vi "Teleop.vi"(10 "Match Info":T2={"Autonomous Elapsed Seconds"=0.0, "TeleOp Elapsed Seconds"=0.0, "Disabled Elapsed Seconds"=0.0, "Visited Autonomous"=FALSE, "Visited TeleOp"=FALSE, "Visited Disabled"=FALSE, "Autonomous Settings"={"Autonomous Style"=enum."Independent", "VI Refnum"=refnum}}, 11 "Call Context":T3) -> ()   [LabVIEW 2019]
doc: "This VI is called for each TeleOp packet received from the DS where the robot is not disabled. It is often used to read from the joysticks and update I/O or to update setpoints for timed control loops. It should complete and return within 20 milliseconds or it may miss DS packets."
uses:
  <vilib>/Rock Robotics/WPI/DriverStation/WPI_DriverStationDerivedRobotMode.ctl
  <vilib>/Rock Robotics/WPI/DriverStation/WPI_DriverStationMatch Info.ctl
  <vilib>/Rock Robotics/WPI/ThirdParty/Phoenix-LabVIEW/Motor Controller/Controls/CTRE_Phoenix_MotorControl_ControlMode.ctl
  <vilib>/Rock Robotics/WPI/Utilities/WPI_GetSetVariantRefNum.vi
  <vilib>/Rock Robotics/Network Tables/NT Write Boolean Array.vi
  <vilib>/Rock Robotics/Network Tables/NT Write Numeric Array.vi
  <vilib>/Rock Robotics/Network Tables/NT Read Boolean.vi
  <vilib>/Rock Robotics/Network Tables/NT Read Number.vi
  <vilib>/Rock Robotics/WPI/ThirdParty/Phoenix-LabVIEW/Motor Controller/Get/CTRE_Phoenix_MotorController_IntegratedSensorData_TalonFX.vi
  <vilib>/Rock Robotics/WPI/ThirdParty/Phoenix-LabVIEW/Motor Controller/Get/CTRE_Phoenix_MotorController_GetVoltage.vi
  <vilib>/Rock Robotics/WPI/ThirdParty/Phoenix-LabVIEW/Motor Controller/Get/CTRE_Phoenix_MotorController_GetSelectedSensorData.vi
  <vilib>/Rock Robotics/WPI/ThirdParty/Phoenix-LabVIEW/Motor Controller/Get/CTRE_Phoenix_MotorController_GetSupplyAndStatorCurrent_Enhanced.vi
  <vilib>/Rock Robotics/WPI/ThirdParty/Phoenix-LabVIEW/Motor Controller/Get/CTRE_Phoenix_MotorController_GetTemperature.vi
  <vilib>/Rock Robotics/Network Tables/NT Write Number.vi
  <vilib>/Rock Robotics/Network Tables/NT Write Boolean.vi
  Global 2.vi
  <vilib>/addons/control/pid/NI_PID_pid.lvlib
  <vilib>/addons/control/pid/pid.llb/PID (DBL).vi
panel:
  in  "Acc Voltage":dbl=0.5
  in  "DriveScale":dbl(slide)=0.7556179775280899 min=0.25 max=1.0 step=0.1 scale=0.25..1.0
  in  "Steering Scale":dbl(slide)=0.6418539325842696 min=0.25 max=1.0 step=0.1 scale=0.25..1.0
  in  "channel name(s) in (Untitled)":string[](array[string])
  in  "group name in (Untitled)":string="Velocity Data"
  in  "PID gains":T1={"proportional gain (Kc)"=1.0, "integral time (Ti, min)"=0.01, "derivative time (Td, min)"=0.0} {"derivative time (Td, min)" format="%.3f"; "integral time (Ti, min)" format="%.3f"; "proportional gain (Kc)" format="%.3f"}
  out "Horizontal Angle":dbl
  out "Waveform Chart":i32(graph)
  in  "Output":dbl=17250.0
  out "Output Voltage":dbl
  out "Bus Voltage":dbl
  out "Percent Output":dbl
  out "Velocity (Raw Sensor Units per 100 ms)":i32
  out "Position (Raw Sensor Units)":i32
  out "Stator Current":dbl
  out "Supply Current":dbl
  out "Absolute Position":dbl
  out "Velocity":dbl format="%.2f"
  out "Position":dbl format="%.2f"
  out "Sample Slider 0":dbl(slide) scale=0.0..5.0
  out "Sample Boolean 1":bool
  out "Sample Boolean 0":bool
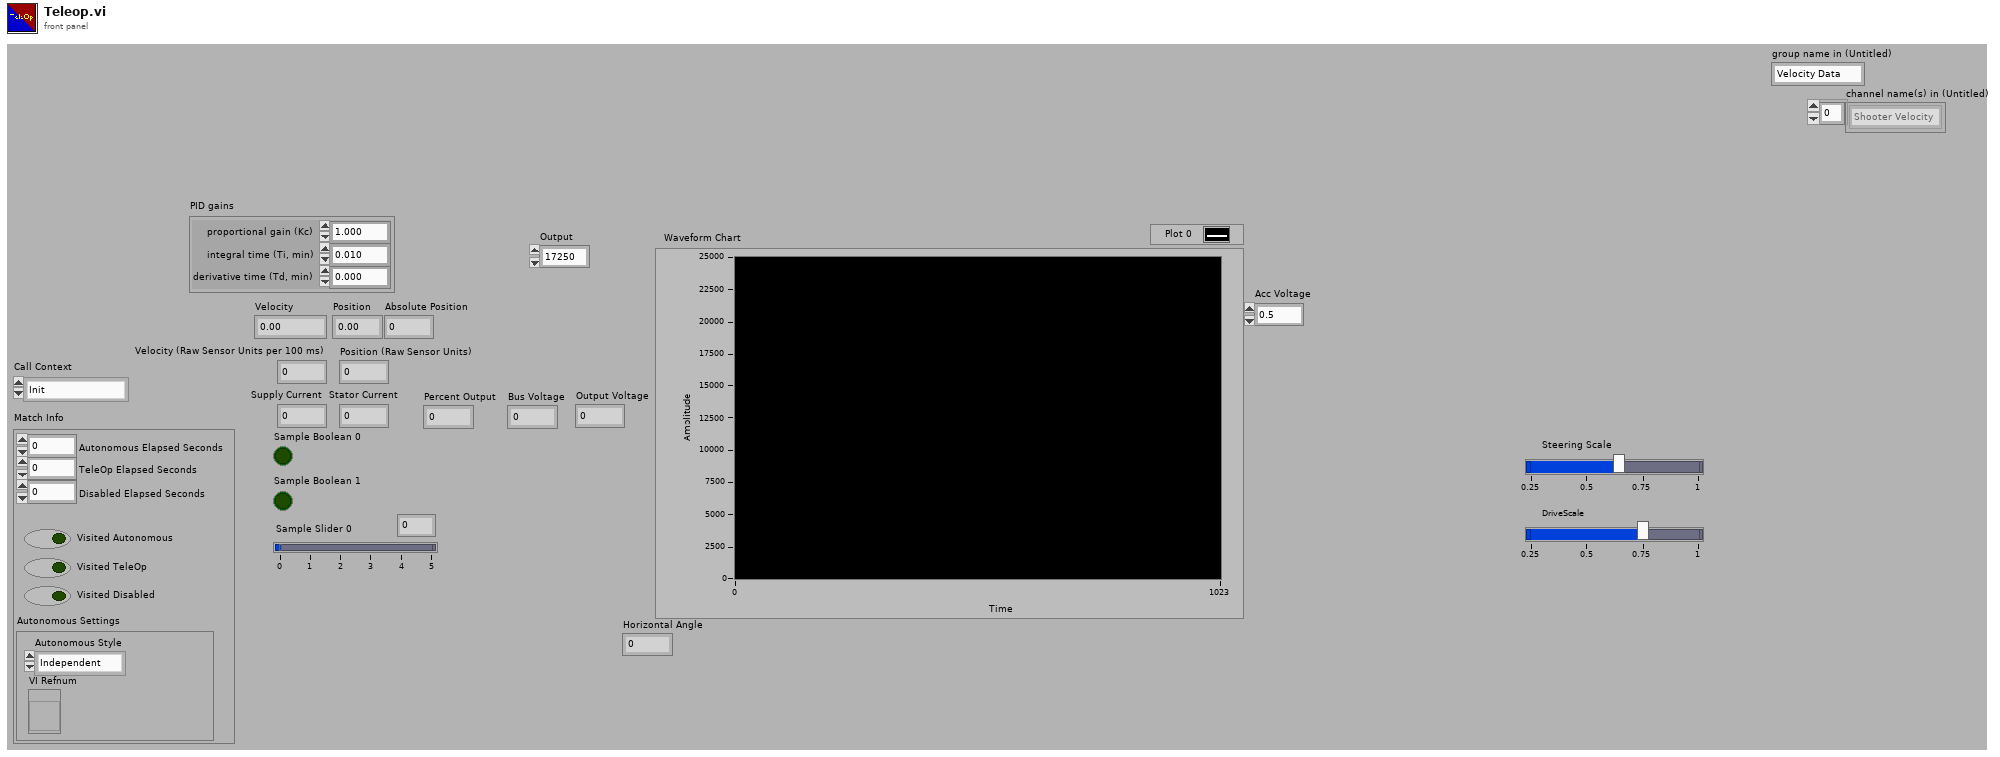
[diagram p1: front panel]
types:
  T1 = cluster{"proportional gain (Kc)":dbl, "integral time (Ti, min)":dbl, "derivative time (Td, min)":dbl}
  T2 = typedef "WPI_DriverStationMatch Info.ctl" = cluster{"Autonomous Elapsed Seconds":dbl, "TeleOp Elapsed Seconds":dbl, "Disabled Elapsed Seconds":dbl, "Visited Autonomous":bool, "Visited TeleOp":bool, "Visited Disabled":bool, "Autonomous Settings":cluster{"Autonomous Style":enum16{"Iterative", "Independent"}, "VI Refnum":refnum<vi>}}
  T3 = typedef "WPI_DriverStationDerivedRobotMode.ctl" = enum16{"Init", "Execute", "Stop"}
  T4 = typedef "CTRE_Phoenix_MotorControl_ControlMode.ctl" = u16
  T5 = typedef "WPI_JoystickDevRef.ctl" = cluster{"Device":T6}
  T6 = typedef "WPI_JoystickDeviceEnum.ctl" = enum16{"USB 0", "USB 1", "USB 2", "USB 3", "USB 4", "USB 5"}
  T7 = cluster{"Axes[0]":dbl, "Axes[1]":dbl, "Axes[2]":dbl, "Axes[3]":dbl, "Axes[4]":dbl, "Axes[5]":dbl, "Axes[6]":dbl, "Axes[7]":dbl, "Axes[8]":dbl}
  T8 = typedef "WPI_MotorControlDeviceRef.ctl" = cluster{"DeviceStatus":errorcluster, "Type":T9, "PWM":cluster{"PWM Channel":T10, "DeadBand":T11}, "CAN":cluster{"Device Number":u8, "SetOutput VI Ref":variant, "GetOutput VI Ref":variant, "Enable VI Ref":variant, "Disable VI Ref":variant, "Data":variant}, "Invert":bool, "DIO PWM":cluster{"PWM \"Enable\" Channel":T10, "DIOChannel":T12, "PWM Rate":dbl}}
  T9 = typedef "WPI_MotorControlType.ctl" = enum16{"PWM", "CAN", "DIO PWM"}
  T10 = typedef "FPGA_DIOPWMChannel.ctl" = enum8{"PWM 0", "PWM 1", "PWM 2", "PWM 3", "PWM 4", "PWM 5", "PWM 6", "PWM 7", "PWM 8", "PWM 9", "PWM MXP 0", "PWM MXP 1", "PWM MXP 2", "PWM MXP 3", "PWM MXP 4", "PWM MXP 5", "PWM MXP 6", "PWM MXP 7", "PWM MXP 8", "PWM MXP 9", "Invalid"}
  T11 = typedef "WPI_PWMDeadband.ctl" = cluster{"Name":string, "maxPositivePwm":i32, "minPositivePwm":i32, "centerPwm":i32, "maxNegativePwm":i32, "minNegativePwm":i32, "angularRange":u16}
  T12 = typedef "FPGA_DIOChannel.ctl" = enum8{"DIO 0", "DIO 1", "DIO 2", "DIO 3", "DIO 4", "DIO 5", "DIO 6", "DIO 7", "DIO 8", "DIO 9", "DIO MXP 0", "DIO MXP 1", "DIO MXP 2", "DIO MXP 3", "DIO MXP 4", "DIO MXP 5", "DIO MXP 6", "DIO MXP 7", "DIO MXP 8", "DIO MXP 9", "DIO MXP 10", "DIO MXP 11", "DIO MXP 12", "DIO MXP 13", "DIO MXP 14", "DIO MXP 15", "SPI Port CS1", "SPI Port CS2", "SPI Port CS3", "SPI Port MISO", "SPI Port MOSI", "Invalid"}
  T13 = cluster{"Buttons[0]":bool, "Buttons[1]":bool, "Buttons[2]":bool, "Buttons[3]":bool, "Buttons[4]":bool, "Buttons[5]":bool, "Buttons[6]":bool, "Buttons[7]":bool, "Buttons[8]":bool}
  T14 = typedef "WPI_RobotDriveDevRef.ctl" = cluster{"DevStatus":errorcluster, "Motors[]":T8[], "Square Inputs":bool, "Max Output":dbl}
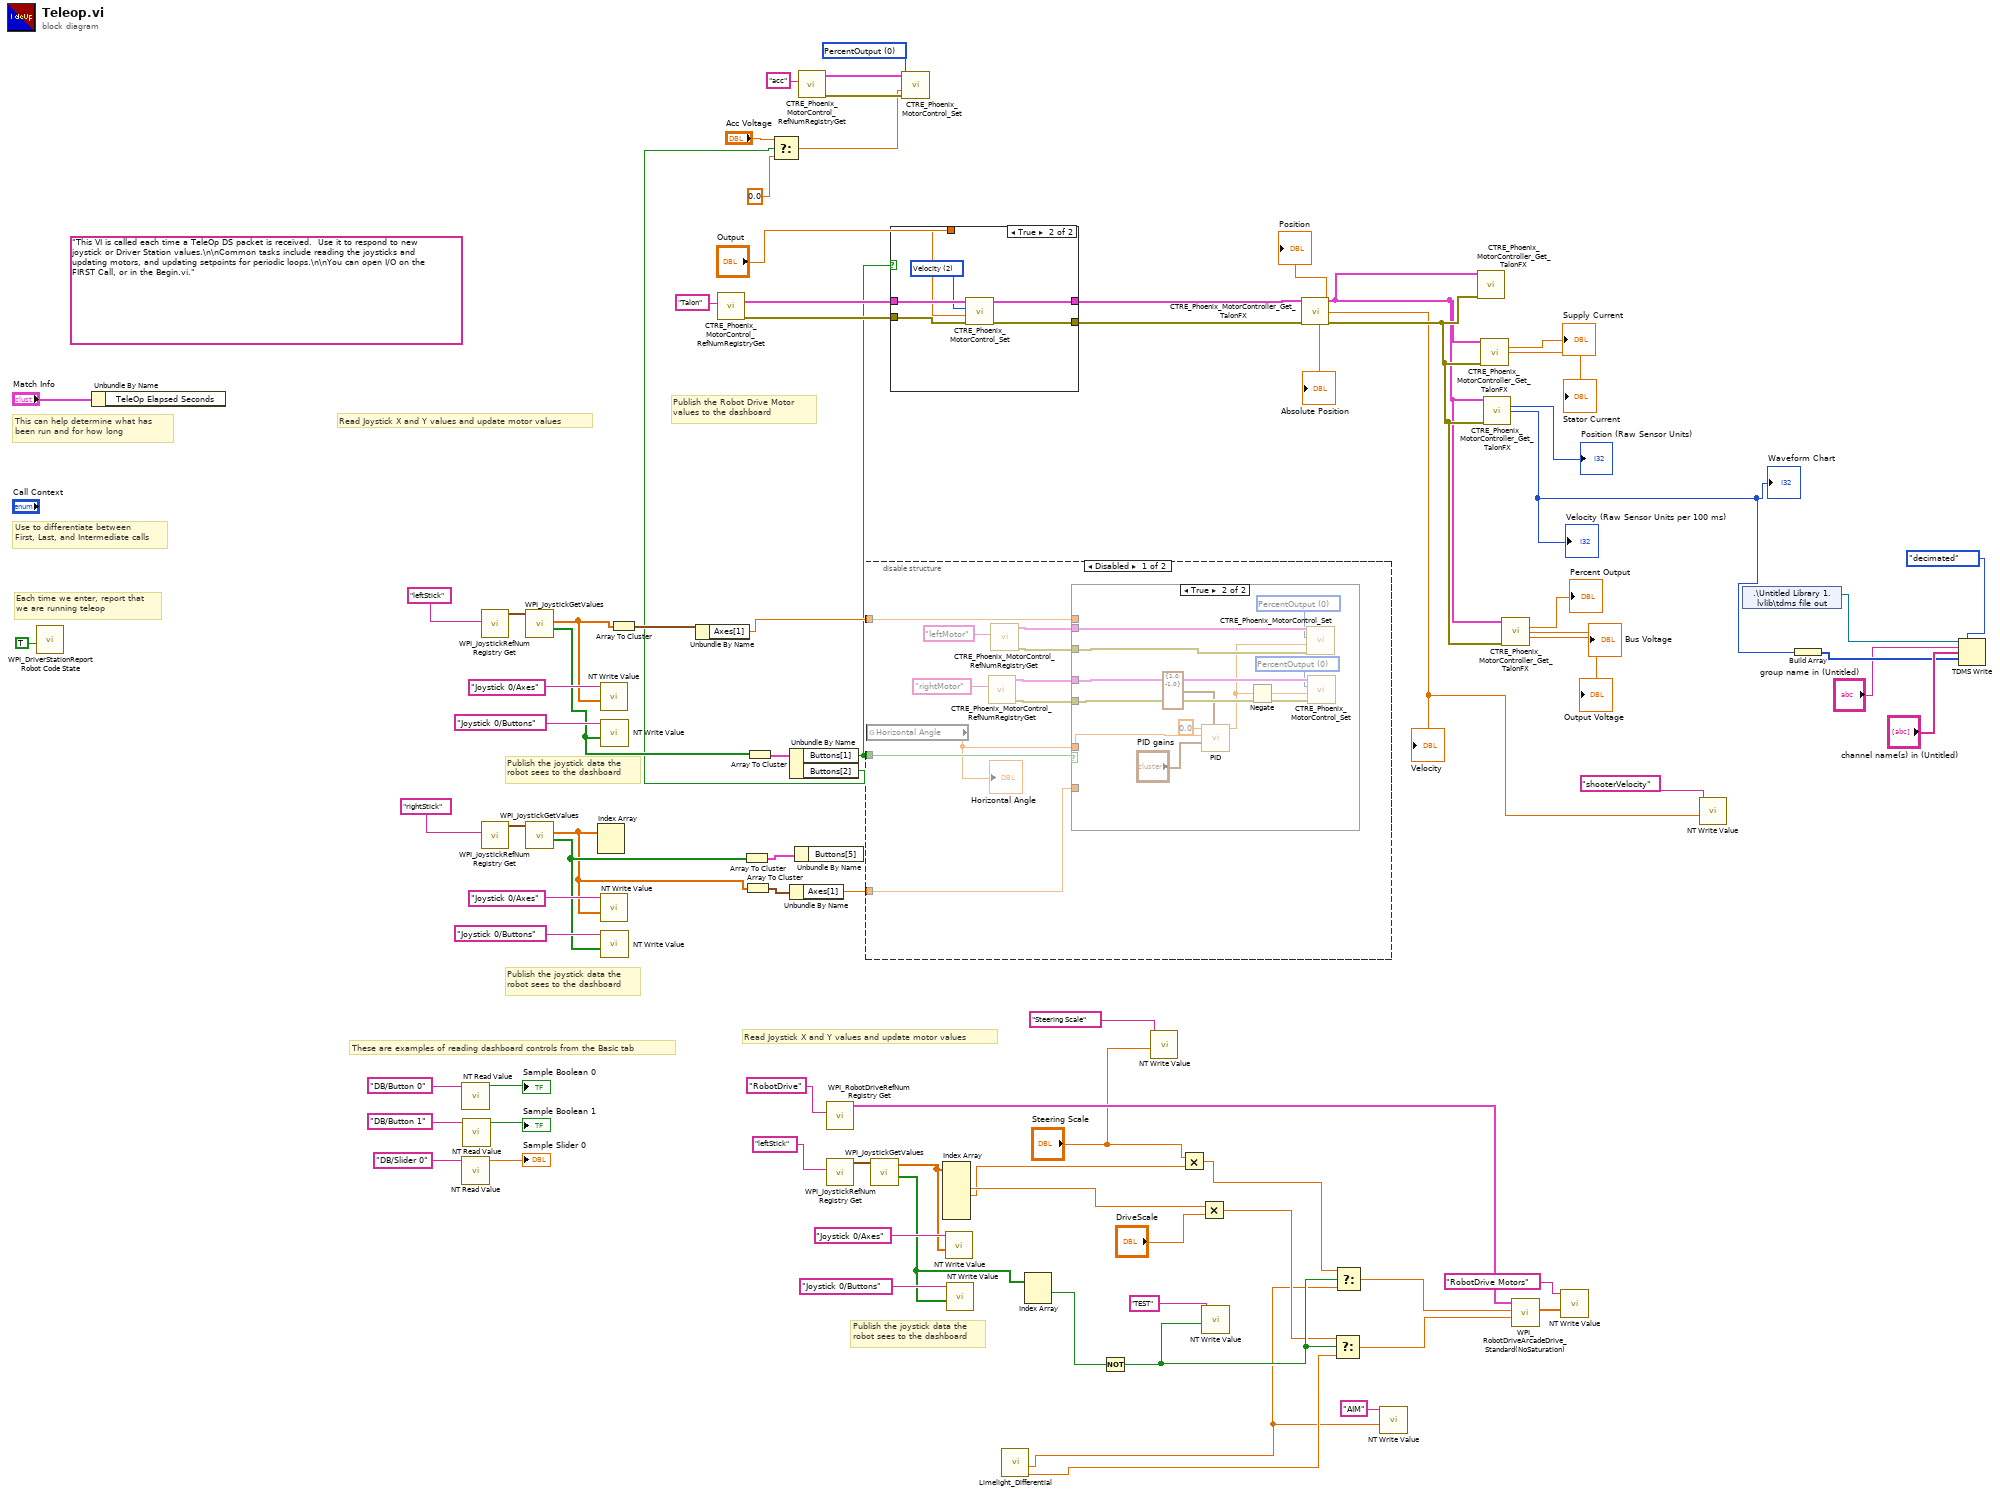
[diagram p0: block diagram]
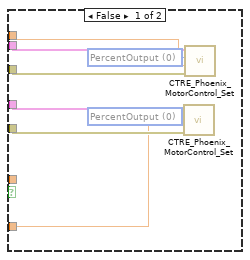
[diagram p2: hidden frame]
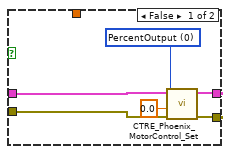
[diagram p4: hidden frame]
diagram:
  w6 = T4 0 items=["PercentOutput"=0, "Position"=1, "Velocity"=2, "Current"=3, "Follower"=5, "MotionProfile"=6, "MotionMagic"=7, "MotionProfileArc"=10, "Disabled"=15] ("Control Mode")
  (unwired) "This VI is called each time a TeleOp DS packet is received.  Use it to respond to new joystick or Driver Station values.\n\nCommon tasks include reading the joysticks and updating motors, and updating setpoints for periodic loops.\n\nYou can open I/O on the FIRST Call, or in the Begin.vi."
  # "Publish the joystick data the\nrobot sees to the dashboard"
  # "Read Joystick X and Y values and update motor values"
  # "Publish the joystick data the\nrobot sees to the dashboard"
  # "These are examples of reading dashboard controls from the Basic tab"
  # "Publish the Robot Drive Motor\nvalues to the dashboard"
  # "Publish the joystick data the\nrobot sees to the dashboard"
  # "Each time we enter, report that\nwe are running teleop"
  # "Use to differentiate between\nFirst, Last, and Intermediate calls"
  # "This can help determine what has\nbeen run and for how long"
  # "Read Joystick X and Y values and update motor values"
  n1 = call <vilib>:"WPI_DriverStationReport Robot Code State.vi"("TeleOp"=TRUE ("Autonomous")) -> ()  [unwired: 10 in, 1 out]
  n2 = Unbundle By Name("Match Info") -> ()  [unwired: 1 out]
  n3 = call-poly <vilib>:"NT Read Value.vi"("Name"="DB/Button 0" ("refnum name")) -> ("Boolean"=→"Sample Boolean 0":bool)  [unwired: 9 in, 1 out]
  n4 = call-poly <vilib>:"NT Read Value.vi"("Name"="DB/Slider 0" ("refnum name")) -> ("Numeric"=→"Sample Slider 0":dbl)  [unwired: 9 in, 1 out]
  n5 = call-poly <vilib>:"NT Read Value.vi"("Name"="DB/Button 1" ("refnum name")) -> ("Boolean"=→"Sample Boolean 1":bool)  [unwired: 9 in, 1 out]
  n6 = call <vilib>:"WPI_JoystickRefNum Registry Get.vi"("refnum name"="leftStick") -> ("JoystickDevRef"=w82:T5)  [unwired: 1 in, 9 out]
  n7 = call <vilib>:"WPI_JoystickRefNum Registry Get.vi"("refnum name"="rightStick") -> ("JoystickDevRef"=w55:T5)  [unwired: 1 in, 9 out]
  n8 = call <vilib>:"WPI_JoystickGetValues.vi"("JoystickDevRef"=w82) -> ("Buttons"=w52:bool[], "Axes"=w50:dbl[])  [unwired: 6 in, 3 out]
  n9 = call <vilib>:"WPI_JoystickGetValues.vi"("JoystickDevRef"=w55) -> ("Buttons"=w49:bool[], "Axes"=w45:dbl[])  [unwired: 6 in, 3 out]
  n10 = Index Array(array=w45) -> ()  [unwired: 2 in, 2 out]
  n11 = call-poly <vilib>:"NT Write Value.vi"("Numeric Array"=w50, "Name"="Joystick 0/Axes") -> ()  [unwired: 9 in, 1 out]
  n12 = call-poly <vilib>:"NT Write Value.vi"("Numeric Array"=w45, "Name"="Joystick 0/Axes") -> ()  [unwired: 9 in, 1 out]
  n13 = call-poly <vilib>:"NT Write Value.vi"("Boolean Array"=w52, "Name"="Joystick 0/Buttons") -> ()  [unwired: 9 in, 1 out]
  n14 = call-poly <vilib>:"NT Write Value.vi"("Boolean Array"=w49, "Name"="Joystick 0/Buttons") -> ()  [unwired: 9 in, 1 out]
  n15 = Array To Cluster(array=w50) -> (cluster=w47:T7)
  n16 = Unbundle By Name(w47) -> ("Axes[1]"=w46:dbl)
  n17 = call <vilib>:"CTRE_Phoenix_MotorControl_RefNumRegistryGet.vi"("refnum name"="Talon") -> ("error out"=w71:errorcluster, "PhoenixMotorControlDevRef"=w72:T8)  [unwired: 9 in]
  n18 = Array To Cluster(array=w49) -> (cluster=w48:T13)
  n19 = Array To Cluster(array=w45) -> (cluster=w44:T7)
  n20 = Array To Cluster(array=w52) -> (cluster=w51:T13)
  n21 = Unbundle By Name(w51) -> ("Buttons[1]"=w10:bool, "Buttons[2]"=w1:bool)
  n22 = Select(t="Acc Voltage", s=w1, f=0.0) -> (s? t:f=w4:dbl)
  n23 = Unbundle By Name(w44) -> ("Axes[1]"=w43:dbl)
  n24 = Unbundle By Name(w48) -> ()  [unwired: 1 out]
  n25 = call <vilib>:"CTRE_Phoenix_MotorControl_RefNumRegistryGet.vi"("refnum name"="acc") -> ("error out"=w7:errorcluster, "PhoenixMotorControlDevRef"=w8:T8)  [unwired: 9 in]
  n26 = call <vilib>:"WPI_RobotDriveRefNum Registry Get.vi"("refnum name"="RobotDrive") -> ("RobotDriveDevRef"=w33:T14)  [unwired: 1 in, 9 out]
  n27 = call <vilib>:"WPI_JoystickRefNum Registry Get.vi"("refnum name"="leftStick") -> ("JoystickDevRef"=w31:T5)  [unwired: 1 in, 9 out]
  n28 = disable-structure shown="Disabled" {
    disable-tunnel: w10 -> [w92 _]
    disable-tunnel: w46 -> [w87 _]
    disable-tunnel: w43 -> [w86 _]
    frame Disabled {
      n29 = global read "Global 2.vi" "Horizontal Angle"() -> (w85:dbl)
      "Horizontal Angle" <- w85
      n30 = call <vilib>:"CTRE_Phoenix_MotorControl_RefNumRegistryGet.vi"("refnum name"="rightMotor") -> ("error out"=w88:errorcluster, "PhoenixMotorControlDevRef"=w89:T8)  [unwired: 9 in]
      n31 = call <vilib>:"CTRE_Phoenix_MotorControl_RefNumRegistryGet.vi"("refnum name"="leftMotor") -> ("error out"=w90:errorcluster, "PhoenixMotorControlDevRef"=w91:T8)  [unwired: 9 in]
      n32 = case shown="True" w92 {
        tunnel: w91 -> [w102 w112]
        tunnel: w90 -> [w101 w114]
        tunnel: w89 -> [w100 w113]
        tunnel: w88 -> [w99 w111]
        tunnel: w87 -> [w98 _]
        tunnel: w86 -> [w97 _]
        tunnel: w85 -> [_ w106]
        frame False {
          w95 = T4 0 items=["PercentOutput"=0, "Position"=1, "Velocity"=2, "Current"=3, "Follower"=5, "MotionProfile"=6, "MotionMagic"=7, "MotionProfileArc"=10, "Disabled"=15] ("Control Mode")
          w96 = T4 0 items=["PercentOutput"=0, "Position"=1, "Velocity"=2, "Current"=3, "Follower"=5, "MotionProfile"=6, "MotionMagic"=7, "MotionProfileArc"=10, "Disabled"=15] ("Control Mode")
          n33 = call <vilib>:"CTRE_Phoenix_MotorControl_Set.vi"("error in (no error)"=w99, "Output"=w97, "Control Mode"=w96, "PhoenixMotorControlDevRef"=w100) -> ()  [unwired: 6 in, 2 out]
          n34 = call <vilib>:"CTRE_Phoenix_MotorControl_Set.vi"("error in (no error)"=w101, "Output"=w98, "Control Mode"=w95, "PhoenixMotorControlDevRef"=w102) -> ()  [unwired: 6 in, 2 out]
        }
        frame True {
          w109 = T4 0 items=["PercentOutput"=0, "Position"=1, "Velocity"=2, "Current"=3, "Follower"=5, "MotionProfile"=6, "MotionMagic"=7, "MotionProfileArc"=10, "Disabled"=15] ("Control Mode")
          w110 = T4 0 items=["PercentOutput"=0, "Position"=1, "Velocity"=2, "Current"=3, "Follower"=5, "MotionProfile"=6, "MotionMagic"=7, "MotionProfileArc"=10, "Disabled"=15] ("Control Mode")
          n35 = call-poly <vilib>:"PID.vi"("output range"=cluster{"output high":dbl, "output low":dbl} {"output high"=1.0, "output low"=-1.0}, "PID gains"="PID gains", "process variable"=w106, "setpoint"=0.0) -> ("output"=w104:dbl)  [unwired: 6 in, 1 out]
          n36 = Negate(x=w104) -> (-x=w103:dbl)
          n37 = call <vilib>:"CTRE_Phoenix_MotorControl_Set.vi"("error in (no error)"=w114, "Output"=w104, "Control Mode"=w110, "PhoenixMotorControlDevRef"=w112) -> ()  [unwired: 6 in, 2 out]
          n38 = call <vilib>:"CTRE_Phoenix_MotorControl_Set.vi"("error in (no error)"=w111, "Output"=w103, "Control Mode"=w109, "PhoenixMotorControlDevRef"=w113) -> ()  [unwired: 6 in, 2 out]
        }
      }
    }
    frame Enabled {
    }
  }
  n39 = call <vilib>:"WPI_JoystickGetValues.vi"("JoystickDevRef"=w31) -> ("Buttons"=w25:bool[], "Axes"=w28:dbl[])  [unwired: 6 in, 3 out]
  n40 = case shown="True" w10 {
    tunnel: w72 -> [w120 w126]
    tunnel: w71 -> [w119 w125]
    tunnel: [w116 w124] -> w69
    tunnel: [w115 w123] -> w68
    tunnel: "Output" -> [_ w121]
    frame False {
      w118 = T4 0 items=["PercentOutput"=0, "Position"=1, "Velocity"=2, "Current"=3, "Follower"=5, "MotionProfile"=6, "MotionMagic"=7, "MotionProfileArc"=10, "Disabled"=15] ("Control Mode")
      n41 = call <vilib>:"CTRE_Phoenix_MotorControl_Set.vi"("error in (no error)"=w119, "Output"=0.0, "Control Mode"=w118, "PhoenixMotorControlDevRef"=w120) -> ("error out"=w115:errorcluster, "PhoenixMotorControlDevRef"=w116:T8)  [unwired: 6 in]
    }
    frame True {
      w122 = T4 2 items=["PercentOutput"=0, "Position"=1, "Velocity"=2, "Current"=3, "Follower"=5, "MotionProfile"=6, "MotionMagic"=7, "MotionProfileArc"=10, "Disabled"=15] ("Control Mode")
      n42 = call <vilib>:"CTRE_Phoenix_MotorControl_Set.vi"("error in (no error)"=w125, "Output"=w121, "Control Mode"=w122, "PhoenixMotorControlDevRef"=w126) -> ("error out"=w123:errorcluster, "PhoenixMotorControlDevRef"=w124:T8)  [unwired: 6 in]
    }
  }
  n43 = call <vilib>:"CTRE_Phoenix_MotorControl_Set.vi"("error in (no error)"=w7, "Output"=w4, "Control Mode"=w6, "PhoenixMotorControlDevRef"=w8) -> ()  [unwired: 6 in, 2 out]
  n44 = Index Array(array=w28) -> (element #2=w17:dbl, element #3=w9:dbl)  [unwired: 6 in, 4 out]
  n45 = call-poly <vilib>:"NT Write Value.vi"("Numeric Array"=w28, "Name"="Joystick 0/Axes") -> ()  [unwired: 9 in, 1 out]
  n46 = call-poly <vilib>:"NT Write Value.vi"("Boolean Array"=w25, "Name"="Joystick 0/Buttons") -> ()  [unwired: 9 in, 1 out]
  n47 = call "Limelight_Differential.vi"() -> ("DriveCommand"=w12:dbl, "SteerCommand"=w11:dbl)  [unwired: 8 in, 1 out]
  n48 = Index Array(array=w25) -> (element #1=w19:bool)  [unwired: 2 in, 1 out]
  n49 = Not(x=w19) -> (.not. x?=w20:bool)
  n50 = call-poly <vilib>:"NT Write Value.vi"("Numeric"="Steering Scale", "Name"="Steering Scale") -> ()  [unwired: 9 in, 1 out]
  n51 = Multiply(x="Steering Scale", y=w9) -> (x*y=w18:dbl)
  n52 = Multiply(x=w17, y="DriveScale") -> (x*y=w15:dbl)
  n53 = call-poly <vilib>:"NT Write Value.vi"("Boolean"=w20, "Name"="TEST") -> ()  [unwired: 9 in, 1 out]
  n54 = call-poly <vilib>:"CTRE_Phoenix_MotorController_Get_TalonFX.vi"("PhoenixMotorControlDevRef"=w69, "error in"=w68) -> ("PhoenixMotorControlDevRef"=w61:T8, "Position"=→"Position":dbl, "Velocity"=w39:dbl, "Absolute Position"=→"Absolute Position":dbl, "error out"=w62:errorcluster)  [unwired: 9 in]
  "Velocity" <- w39
  n55 = Select(t=w15, s=w20, f=w12) -> (s? t:f=w23:dbl)
  n56 = Select(t=w18, s=w20, f=w11) -> (s? t:f=w24:dbl)
  n57 = call-poly <vilib>:"NT Write Value.vi"("Numeric"=w11, "Name"="AIM") -> ()  [unwired: 9 in, 1 out]
  n58 = call-poly <vilib>:"CTRE_Phoenix_MotorController_Get_TalonFX.vi"("PhoenixMotorControlDevRef"=w61, "error in"=w62) -> ()  [unwired: 11 in, 3 out]
  n59 = call-poly <vilib>:"CTRE_Phoenix_MotorController_Get_TalonFX.vi"("PhoenixMotorControlDevRef"=w61, "error in"=w62) -> ("Supply Current"=→"Supply Current":dbl, "Stator Current"=→"Stator Current":dbl)  [unwired: 10 in, 2 out]
  n60 = call-poly <vilib>:"CTRE_Phoenix_MotorController_Get_TalonFX.vi"("PhoenixMotorControlDevRef"=w61, "error in"=w62) -> ("Position (Raw Sensor Units)"=→"Position (Raw Sensor Units)":i32, "Velocity (Raw Sensor Units per 100 ms)"=w37:i32)  [unwired: 10 in, 2 out]
  "Velocity (Raw Sensor Units per 100 ms)" <- w37
  "Waveform Chart" <- w37
  n61 = call-poly <vilib>:"CTRE_Phoenix_MotorController_Get_TalonFX.vi"("PhoenixMotorControlDevRef"=w61, "error in"=w62) -> ("Percent Output"=→"Percent Output":dbl, "Output Voltage"=→"Output Voltage":dbl, "Bus Voltage"=→"Bus Voltage":dbl)  [unwired: 9 in, 2 out]
  n62 = call <vilib>:"WPI_RobotDriveArcadeDrive_Standard(NoSaturation).vi"("Y axis value"=w23, "X axis value"=w24, "RobotDriveDevRef"=w33) -> ("Motor Values"=w27:dbl[])  [unwired: 1 in, 7 out]
  n63 = call-poly <vilib>:"NT Write Value.vi"("Numeric Array"=w27, "Name"="RobotDrive Motors") -> ()  [unwired: 9 in, 1 out]
  n64 = call-poly <vilib>:"NT Write Value.vi"("Numeric"=w39, "Name"="shooterVelocity") -> ()  [unwired: 9 in, 1 out]
  n65 = shared-variable ".\\Untitled Library 1.lvlib\\tdms file out"() -> (w38:refnum<k34>)  [unwired: 1 in, 1 out]
  n66 = Build Array(w37) -> (w36:i32[])
  n67 = TDMS Write(0:w38, 1:enum16{"decimated", "interleaved"}."decimated" ("data layout (0:decimated)"), 5:"group name in (Untitled)", 7:"channel name(s) in (Untitled)", 9:w36) -> ()  [unwired: 1 in, 4 out]
